vi "Wait for finish.vi"(8 "error in (no error)":errorcluster, 9 "timeout in ms (-1)":i32=-1, 11 "Process In":refnum<class "Debug View.lvclass">) -> (0 "error out":errorcluster, 1 "timed out?":bool, 3 "Process Out":refnum<class "Debug View.lvclass">)   [LabVIEW 2020]
uses:
  Debug View.lvclass
  Debug View.lvclass/Debug View.ctl
  <vilib>/Utility/error.llb/Error Cluster From Error Code.vi
  <vilib>/ErrorRing/Error Ring.xnode
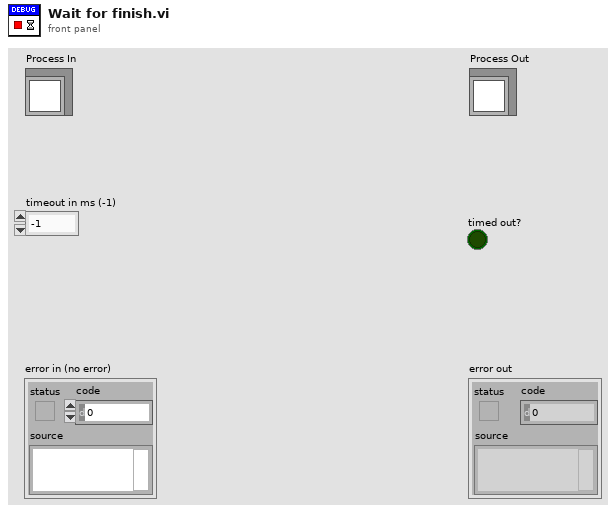
[diagram p1: front panel]
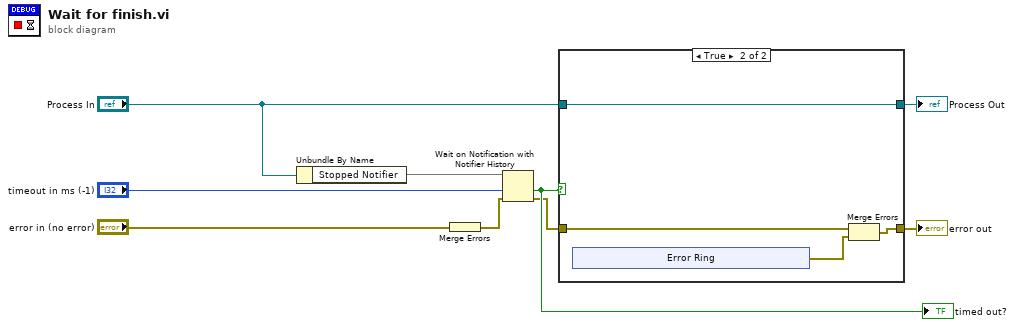
[diagram p0: block diagram]
diagram:
  n1 = Unbundle By Name("Process In") -> ("Stopped Notifier"=w9)
  n2 = Merge Errors("error in (no error)") -> (w1:errorcluster)
  n3 = Wait on Notification with Notifier History(0:w9, 2:"timeout in ms (-1)", 3:w1) -> (10:w5:bool, 11:w4:errorcluster)  [unwired: 1 in, 2 out]
  "timed out?" <- w5
  n4 = case shown="True" w5 {
    tunnel: [w10 w13] -> w6
    tunnel: w4 -> [w10 w14]
    tunnel: [w11 w15] -> w3
    tunnel: "Process In" -> [w11 w15]
    frame False {
    }
    frame True {
      n5 = xnode "Error Ring"() -> ("error out"=w12:errorcluster)
      n6 = Merge Errors(w14, w12) -> (w13:errorcluster)
    }
  }
  "error out" <- w6
  "Process Out" <- w3
